vi "FGV_ARCH_AUDIT_EDITOR_records_display.vi"(4 "front_panel_reference":refnum<vi>, 6 "SQL_listbox_reference":refnum<vi>, 7 "options":T3, 8 "error_in":errorcluster, 10 "uneditable_columns":string[](array[string])=["ID", "CREATION_TIME", "CREATED_BY"], 11 "input":variant) -> (0 "error_out":errorcluster, 1 "all_info":T1, 2 "array_param_output":string[](array[string]), 3 "string_param_output":string)   [LabVIEW 2020]
uses:
  FGV_ARCH_AUDIT_EDITOR_records_display.ctl
  ARCH_AUDIT_EDITOR_all_info.ctl
  MAIN/SQL_record_states.ctl
  ini/typedef/CLIENT_all_config_info.ctl
  ini/typedef/CLIENT_main_ini_file.ctl
  queues/typedef/CLIENT_queue_refnums.ctl
  queues/typedef/SQL_EDITOR_queue_element.ctl
  MAIN/SQL_EDITOR/SQL_EDITOR_sequence_state.ctl
  queues/typedef/CLIENT_SCANNER_queue_element.ctl
  MAIN/SCANNER/SCANNER_sequence_state.ctl
  queues/typedef/CLIENT_REF_CHG_queue_element.ctl
  MAIN/reference_changed_connection/CLIENT_REF_CHG_sequence_state.ctl
  <userlib>/_OpenG.lib/array/array.llb/Filter 1D Array (String)__ogtk.vi
  <userlib>/_OpenG.lib/array/array.llb/Delete Elements from 1D Array (I32)__ogtk.vi
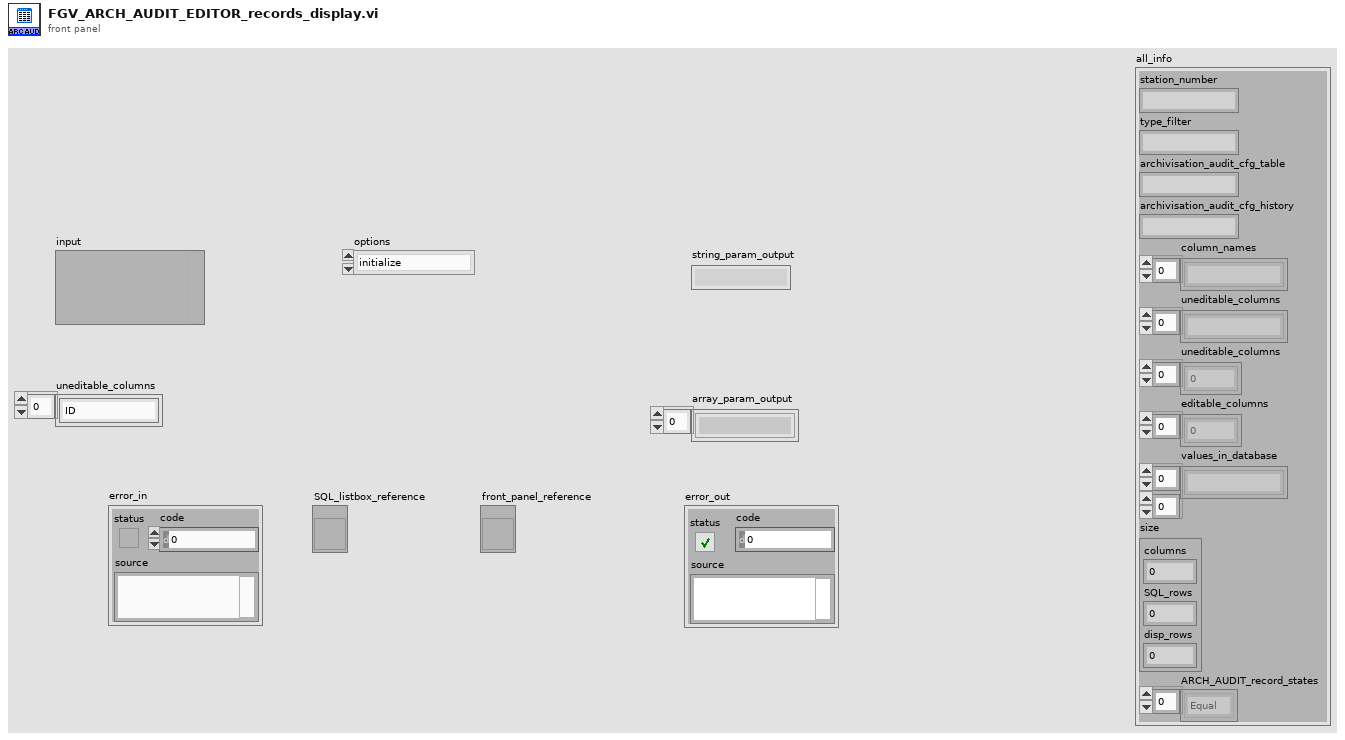
[diagram p1: front panel]
types:
  T1 = typedef "ARCH_AUDIT_EDITOR_all_info.ctl" = cluster{"station_number":string, "type_filter":string, "archivisation_audit_cfg_table":string, "archivisation_audit_cfg_history":string, "column_names":string[], "uneditable_columns":string[], "uneditable_columns":i32[], "editable_columns":i32[], "values_in_database":string[][], "size":cluster{"columns":i32, "SQL_rows":i32, "disp_rows":i32}, "ARCH_AUDIT_record_states":T2[]}
  T2 = typedef "SQL_record_states.ctl" = enum16{"Equal", "Added", "Edited", "Deleted"}
  T3 = typedef "FGV_ARCH_AUDIT_EDITOR_records_display.ctl" = enum16{"initialize", "set_arch_cfg_tables_names", "set_station_number", "set_type_filter", "set_headers", "set_records", "get_arch_cfg_table_name", "get_arch_cfg_hist_table_name", "get_station_number", "get_type_filter", "get_headers", "get_uneditable_columns", "get_all_info", "record_added?", "record_inserted?", "record_edited?", "record_updated?", "record_deleted?", "discard_changes"}
  T4 = typedef "CLIENT_all_config_info.ctl" = cluster{"main_ini_file":T5, "SQL Password":string, "queue_refnums":T6}
  T5 = typedef "CLIENT_main_ini_file.ctl" = cluster{"SQL Driver":string, "SQL Server":string, "SQL Database":string, "SQL UID":string, "Reference table":string, "Reference history":string, "Archivisation CFG table":string, "Archivisation CFG history":string, "Archivisation Audit table":string, "Archivisation Audit history":string, "User table":string, "User history":string, "logout timeout [ms]":i32, "records per page":i32, "default language":string, "REF CHG connection IP":string, "REF CHG remote port":i32, "REF CHG local port":i32, "SCANNER COM port":u16, "SCANNER Baud rate":u32, "SCANNER Data bits":u16, "SCANNER Pairity":enum16{"None", "Odd", "Even", "Mark", "Space"}, "SCANNER Stop bits":u16, "SCANNER Flow control":u16, "SCANNER Termination char":u8}
  T6 = typedef "CLIENT_queue_refnums.ctl" = cluster{"SQL_EDITOR_queue":refnum<queue>, "SCANNER_queue":refnum<queue>, "SCANNER_data":refnum<queue>, "CLIENT_REF_CHG_queue":refnum<queue>}
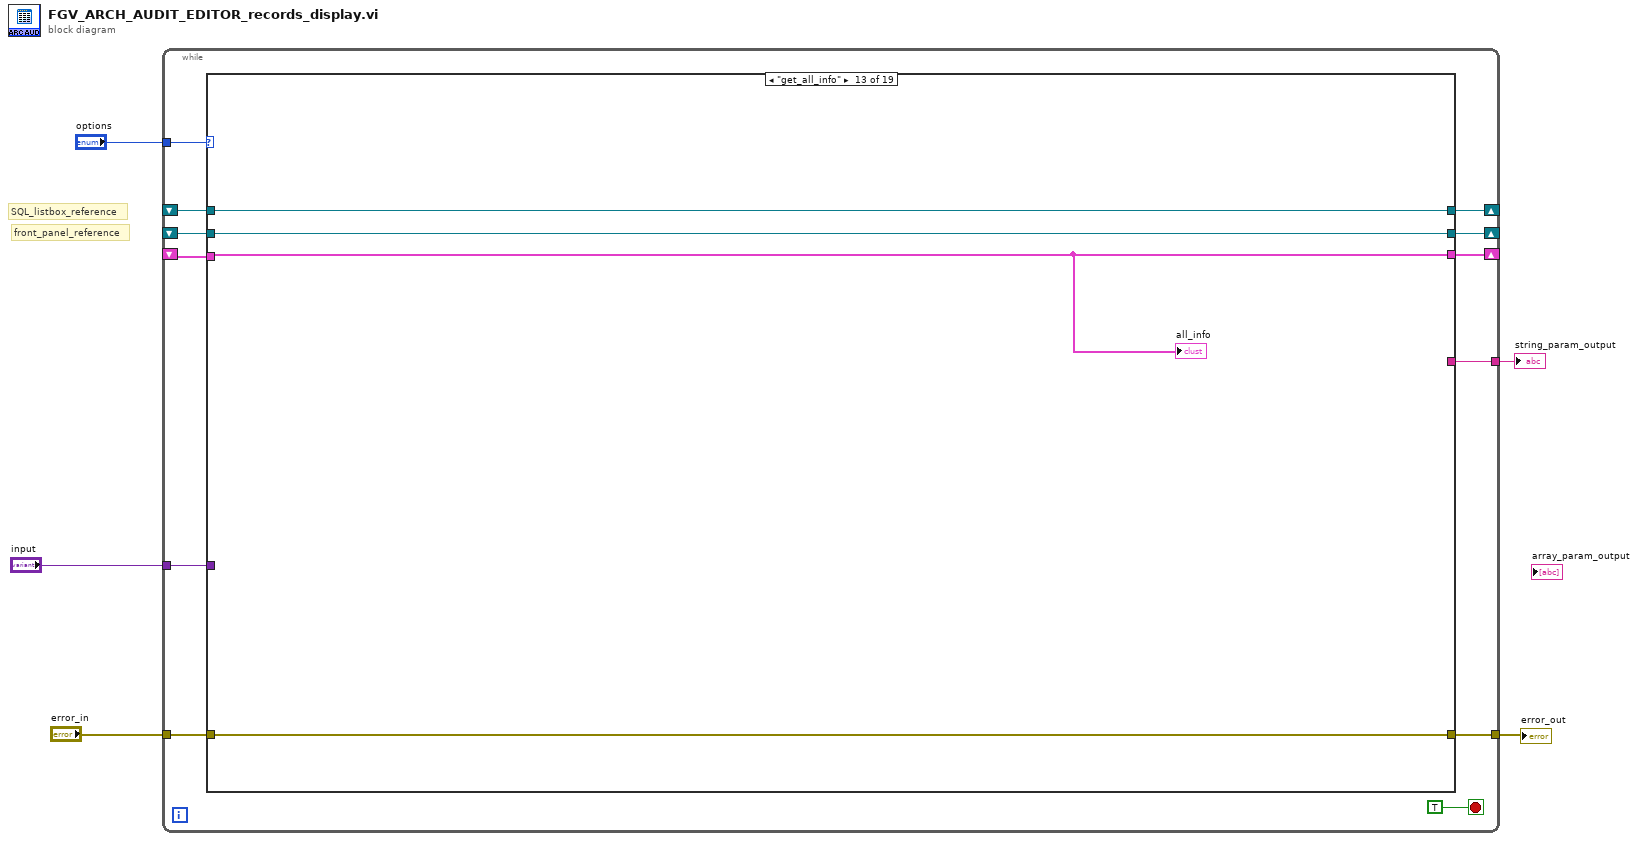
[diagram p0: block diagram]
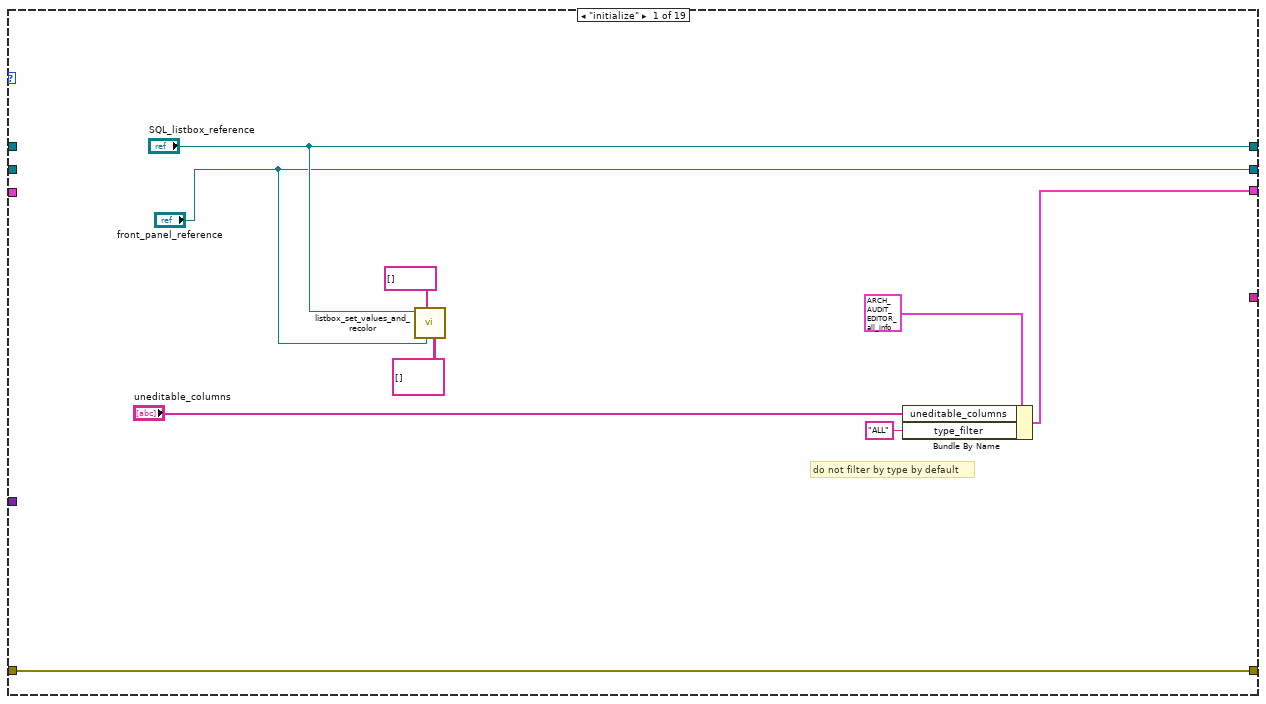
[diagram p2: hidden frame]
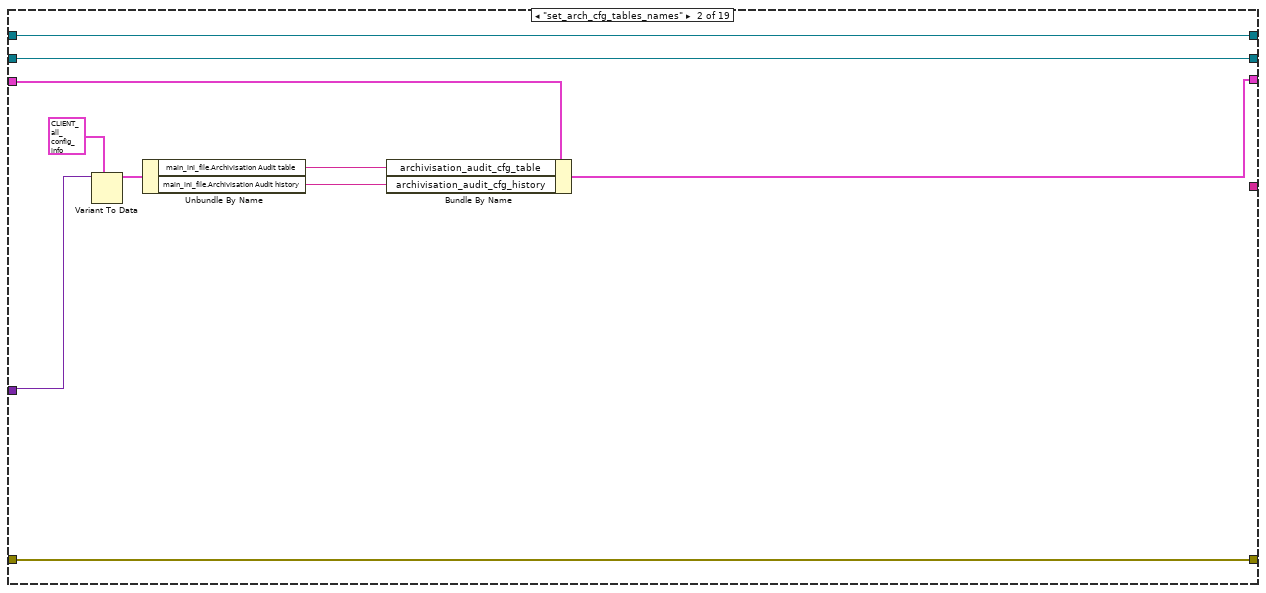
[diagram p3: hidden frame]
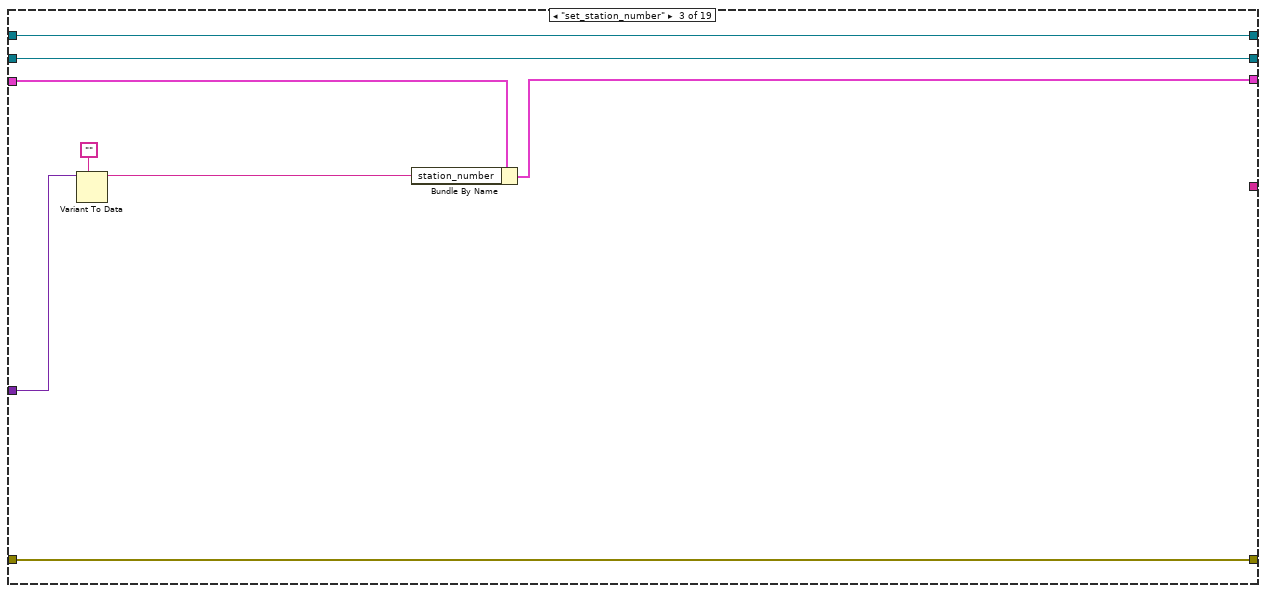
[diagram p4: hidden frame]
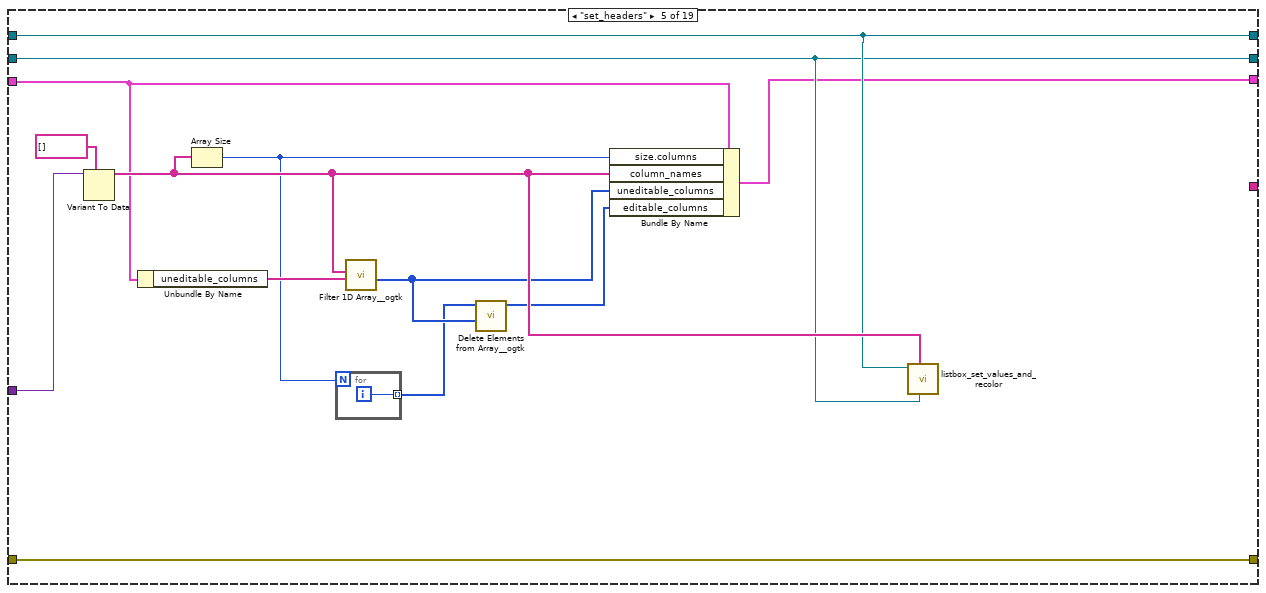
[diagram p6: hidden frame]
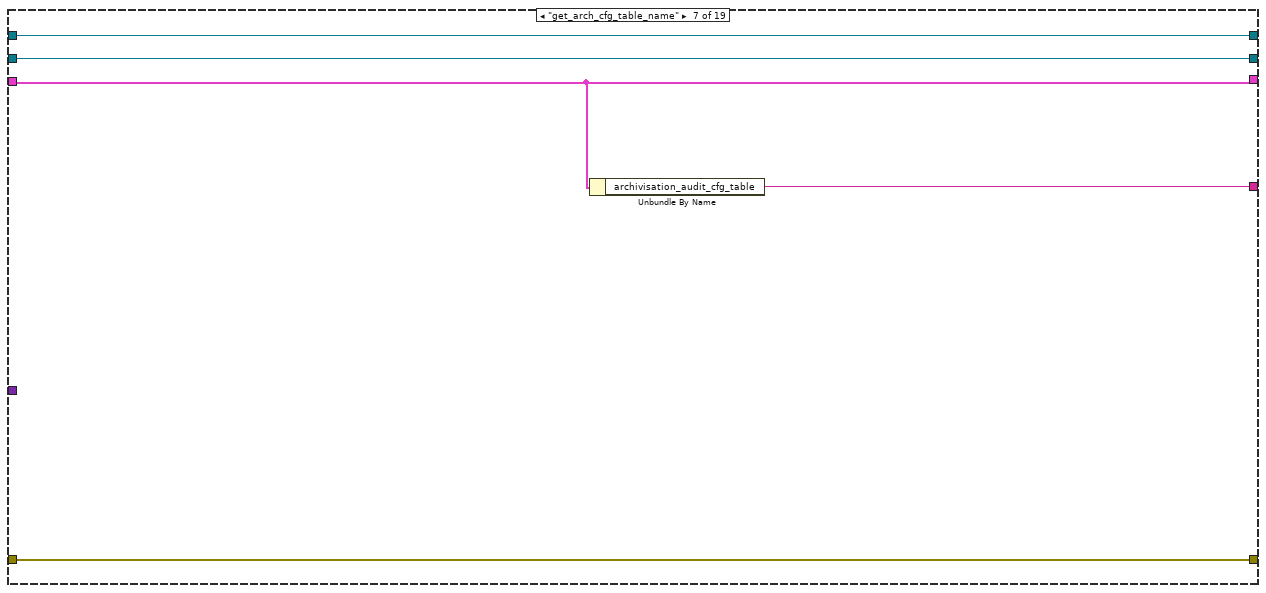
[diagram p8: hidden frame]
diagram:
  # "front_panel_reference"
  # "SQL_listbox_reference"
  n1 = while {
    tunnel: "options" -> [w16]
    shift-right: [w15] -> _
    shift-left: _ -> [w9]
    shift-right: [w14] -> _
    shift-left: _ -> [w8]
    shift-right: [w13] -> _
    shift-left: _ -> [w7]
    tunnel: "error_in" -> [w12]
    tunnel: [w11] -> w3
    tunnel: "input" -> [w10]
    tunnel: [w6] -> w1
    stop <- TRUE stop-if-true
    n2 = case shown="\"get_all_info\"" w16 {
      tunnel: ["SQL_listbox_reference" w36 w44 w47 w51 w64 w69 w72 w75 w78 w81 w84 w88 w91 w94 w97 w100 w103 w106] -> w15
      tunnel: ["front_panel_reference" w35 w43 w46 w50 w63 w68 w71 w74 w77 w80 w83 w87 w90 w93 w96 w99 w102 w105] -> w14
      tunnel: [w20 w27 w37 _ w48 _ w66 _ _ _ _ _ w85 _ _ _ _ _ _] -> w13
      tunnel: w12 -> [w19 w34 w42 w45 w60 w62 w67 w70 w73 w76 w79 w82 w86 w89 w92 w95 w98 w101 w104]
      tunnel: [w19 w34 w42 w45 w60 w62 w67 w70 w73 w76 w79 w82 w86 w89 w92 w95 w98 w101 w104] -> w11
      tunnel: w10 -> [_ w29 w39 _ w52 _ _ _ _ _ _ _ _ _ _ _ _ _ _]
      tunnel: w9 -> [_ w36 w44 w47 w51 w64 w69 w72 w75 w78 w81 w84 w88 w91 w94 w97 w100 w103 w106]
      tunnel: w8 -> [_ w35 w43 w46 w50 w63 w68 w71 w74 w77 w80 w83 w87 w90 w93 w96 w99 w102 w105]
      tunnel: w7 -> [_ w28 w38 _ w49 _ w66 _ _ _ _ _ w85 _ _ _ _ _ _]
      tunnel: [_ _ _ _ _ _ w65 _ _ _ _ _ _ _ _ _ _ _ _] -> w6
      frame "initialize" {
        # "do not filter by type by default"
        n3 = call "listbox_set_values_and_recolor.vi"("item_names"=string[][] [], "front_panel_reference"="front_panel_reference", "column_names"=string[] [], "multicolumn_listbox_reference_in"="SQL_listbox_reference") -> ()  [unwired: 6 in, 2 out]
        n4 = Bundle By Name(cluster=T1 {"station_number"="", "type_filter"="", "archivisation_audit_cfg_table"="", "archivisation_audit_cfg_history"="", "column_names"=[], "uneditable_columns"=[], "uneditable_columns"=[], "editable_columns"=[], "values_in_database"=[], "size"={"columns"=0, "SQL_rows"=0, "disp_rows"=0}, "ARCH_AUDIT_record_states"=[]} ("ARCHIVISATION_AUDIT_all_info"), "uneditable_columns"="uneditable_columns", "type_filter"="ALL") -> (w20:T1)
      }
      frame "set_arch_cfg_tables_names" {
        n5 = Variant To Data(type=T4 {"main_ini_file"={"SQL Driver"="", "SQL Server"="", "SQL Database"="", "SQL UID"="", "Reference table"="", "Reference history"="", "Archivisation CFG table"="", "Archivisation CFG history"="", "Archivisation Audit table"="", "Archivisation Audit history"="", "User table"="", "User history"="", "logout timeout [ms]"=0, "records per page"=0, "default language"="", "REF CHG connection IP"="", "REF CHG remote port"=0, "REF CHG local port"=0, "SCANNER COM port"=0, "SCANNER Baud rate"=0, "SCANNER Data bits"=0, "SCANNER Pairity"=enum."None", "SCANNER Stop bits"=10, "SCANNER Flow control"=0, "SCANNER Termination char"=0}, "SQL Password"="", "queue_refnums"={"SQL_EDITOR_queue"=refnum, "SCANNER_queue"=refnum, "SCANNER_data"=refnum, "CLIENT_REF_CHG_queue"=refnum}} ("all_config_info"), Variant=w29) -> (data=w31:T4)  [unwired: 1 in, 1 out]
        n6 = Unbundle By Name(w31) -> ("main_ini_file.Archivisation Audit table"=w32:string, "main_ini_file.Archivisation Audit history"=w33:string)
        n7 = Bundle By Name(cluster=w28, "archivisation_audit_cfg_table"=w32, "archivisation_audit_cfg_history"=w33) -> (w27:T1)
      }
      frame "set_station_number" {
        n8 = Variant To Data(type="", Variant=w39) -> (data=w40:string)  [unwired: 1 in, 1 out]
        n9 = Bundle By Name(cluster=w38, "station_number"=w40) -> (w37:T1)
      }
      frame "set_type_filter" {
      }
      frame "set_headers" {
        n10 = Variant To Data(type=string[] [], Variant=w52) -> (data=w58:string[])  [unwired: 1 in, 1 out]
        n11 = Unbundle By Name(w49) -> ("uneditable_columns"=w56:string[])
        n12 = Array Size(array=w58) -> (size(s)=w53:i32)
        n13 = for {
          N: w53 -> [_]
          tunnel: [w61] -> w55 mode=indexing
          i -> [w61]
        }
        n14 = call-poly <userlib>:"Filter 1D Array__ogtk.vi"("items to filter"=w56, "array"=w58) -> ("filtered item indices"=w57:i32[])  [unwired: 4 in, 1 out]
        n15 = call-poly <userlib>:"Delete Elements from Array__ogtk.vi"("indices"=w57, "array"=w55) -> ("array w/ subset deleted"=w54:i32[])  [unwired: 8 in, 1 out]
        n16 = Bundle By Name(cluster=w49, "size.columns"=w53, "column_names"=w58, "uneditable_columns"=w57, "editable_columns"=w54) -> (w48:T1)
        n17 = call "listbox_set_values_and_recolor.vi"("front_panel_reference"=w50, "column_names"=w58, "multicolumn_listbox_reference_in"=w51) -> ()  [unwired: 7 in, 2 out]
      }
      frame "set_records" {
      }
      frame "get_arch_cfg_table_name" {
        n18 = Unbundle By Name(w66) -> ("archivisation_audit_cfg_table"=w65:string)
      }
      frame "get_arch_cfg_hist_table_name" {
      }
      frame "get_station_number" {
      }
      frame "get_type_filter" {
      }
      frame "get_headers" {
      }
      frame "get_uneditable_columns" {
      }
      frame "get_all_info" {
        "all_info" <- w85
      }
      frame "record_added?" {
      }
      frame "record_inserted?" {
      }
      frame "record_edited?" {
      }
      frame "record_updated?" {
      }
      frame "record_deleted?" {
      }
      frame "discard_changes" {
      }
    }
  }
  "error_out" <- w3
  "string_param_output" <- w1
